vi "Shutdown.vi"(8 "error in (no error)":errorcluster, 11 "UDP Transceiver in":refnum<class "UDP Transceiver.lvclass">) -> (0 "error out":errorcluster, 3 "UDP Transceiver out":refnum<class "UDP Transceiver.lvclass">)   [LabVIEW 2017, in "UDP.lvlib" / "UDP Transceiver.lvclass"]
uses:
  UDP Transceiver.lvclass
  UDP Transceiver.lvclass/UDP Transceiver.ctl
  Transfer Group Parameters.ctl
  Transfer Group Rx Parameters.ctl
  Transfer Rx Parameters.ctl
  Transfer Group Tx Parameters.ctl
  Transfer Tx Parameters.ctl
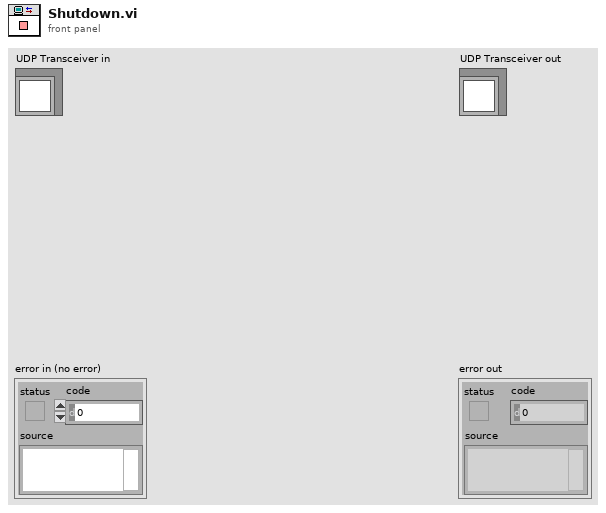
[diagram p1: front panel]
types:
  T1 = typedef "UDP.lvlib/UDP Transceiver.lvclass/Transfer Group Parameters.ctl" = cluster{"Rx":T2, "Tx":T4}
  T2 = typedef "UDP.lvlib/UDP Transceiver.lvclass/Transfer Group Rx Parameters.ctl" = cluster{"Transfers Rx":T3[], "max size":i32}
  T3 = typedef "UDP.lvlib/UDP Transceiver.lvclass/Transfer Rx Parameters.ctl" = cluster{"timeout":i32, "source address":u32, "source port":u16}
  T4 = typedef "UDP.lvlib/UDP Transceiver.lvclass/Transfer Group Tx Parameters.ctl" = cluster{"Transfers Tx":T5[]}
  T5 = typedef "UDP.lvlib/UDP Transceiver.lvclass/Transfer Tx Parameters.ctl" = cluster{"destination port":u16, "destination address":u32}
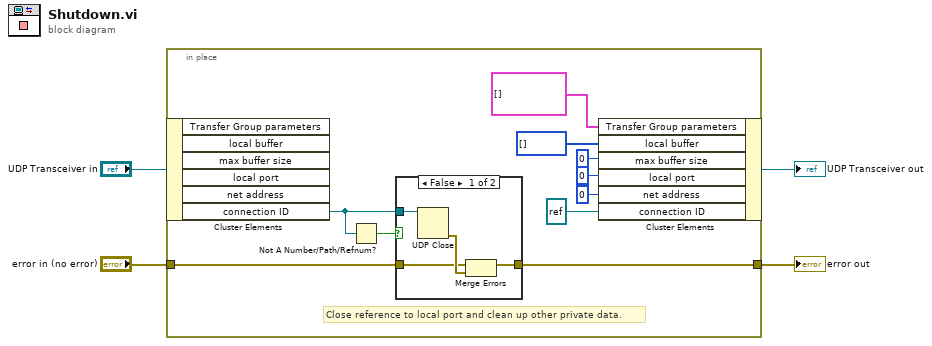
[diagram p0: block diagram]
diagram:
  n1 = in-place {
    in-place-border: "error in (no error)" -> [w14]
    in-place-border: [w13] -> w3
    # "Close reference to local port and clean up other private data."
    n2 = in-place-cluster #1("UDP Transceiver in") -> ("connection ID"=w12:refnum<k16>)  [unwired: 5 out]
    n3 = Not A Number/Path/Refnum?(number/path/refnum=w12) -> (NaN/Path/Refnum?=w11:bool)
    n4 = case shown="False" w11 {
      tunnel: w14 -> [w17 w19]
      tunnel: [w16 w19] -> w13
      tunnel: w12 -> [w15 _]
      frame False {
        n5 = UDP Close(connection ID=w15) -> (error out=w18:errorcluster)  [unwired: 1 in, 1 out]
        n6 = Merge Errors(w17, w18) -> (w16:errorcluster)
      }
      frame True {
      }
    }
    n7 = in-place-cluster #1("Transfer Group parameters"=T1[] [], "local buffer"=u8[] [], "max buffer size"=u64 0, "local port"=u16 0, "net address"=u32 0, "connection ID"=refnum<k16> refnum ("connection ID out")) -> (→"UDP Transceiver out":refnum<class "UDP Transceiver.lvclass">)
  }
  "error out" <- w3
